vi "获取复合步骤名称XPath表达式.vi"(11 "查询参数":string) -> (2 "FlowId":string, 3 "name":string)   [LabVIEW 2016, in "斯坦道总磷.lvlib"]
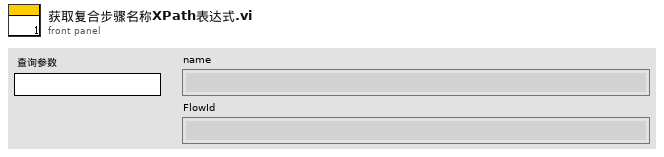
[diagram p1: front panel]
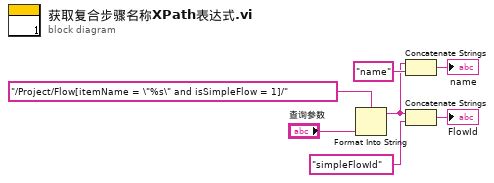
[diagram p0: block diagram]
diagram:
  n1 = Format Into String(format string="/Project/Flow[itemName = \"%s\" and isSimpleFlow = 1]/" ("格式字符串"), "查询参数") -> (resulting string=w3:string)  [unwired: 2 in, 1 out]
  n2 = Concatenate Strings(w3, "name" ("字符串")) -> (→"name":string)
  n3 = Concatenate Strings(w3, "simpleFlowId" ("字符串")) -> (→"FlowId":string)
